vi "TLB Native Dynamic Events ver 0.07D.vi"() -> ()   [LabVIEW 2018]
uses:
  Labview Training Phase 2/Enum Controls/States for Action Engine.ctl
  Type def/TLB event states.ctl
  Type def/TLB MHL States.ctl
  <vilib>/Studica/Studica Toolkit/Background/I2C Channel.ctl
  <vilib>/Studica/Studica Toolkit/NavX/NavX.lvlib
  <vilib>/myRIO/Common/Instrument Driver Framework/myRIO v1.0/AI/typedefs/AI Channels Enum.ctl
  <vilib>/myRIO/Common/Instrument Driver Framework/myRIO v1.0/AI/typedefs/AI Channels List.ctl
  Type def/Type def.ctl
  Type def/Motor Control Cluster.ctl
  <vilib>/Studica/Studica Blackhawk/Blackhawk.lvlib
  <vilib>/Studica/Studica Toolkit/Background/Mxp Selection.ctl
  <vilib>/Studica/Studica Toolkit/Background/DIO Channel.ctl
  <vilib>/NI_Real-Time Target Support.lvlib
  <vilib>/ptbypt/NI_PtbyPt.lvlib
  <vilib>/addons/control/pid/NI_PID_pid.lvlib
  Underlying VI's/Webcam FGV Low level ver/State control.ctl
  <vilib>/userdefined/High Color/IMAQdx.ctl
  <vilib>/addons/control/pid/pid.llb/PID (DBL).vi
panel:
  out "Manual Zero Yaw":bool
  out "BH Loop":i32
  out "NavX Loop":i32
  out "IR Loop":i32
  out "Speed and distance cluster":T1
  out "Cluster":T2
  out "Displacement":T3
  out "Fused Heading":dbl
  in  "error in (no error)":errorcluster
  in  "RED LED State":enum16{"OFF", "ON", "BLINK"}(ring)
  in  "GREEN LED State":enum16{"OFF", "ON", "BLINK"}(ring)
  in  "Red LED":bool
  in  "Green LED":bool
  in  "NavX Zero Yaw":bool
  out "Input state":i8
  out "Waveform Chart 2":dbl(graph)
  out "Waveform Chart":dbl(graph)
  in  "STOP":bool
  out "DIO 0":bool
  out "DIO 1":bool
  out "Limit Switch Array":bool[](array[boolean])
  out "error out":errorcluster
  out "L/R average":fxp<+,64,64>
  out "Right Ultrasonic":fxp<+,64,16>
  out "Left Ultrasonic":fxp<+,64,16>
  out "Right IR Sensor":dbl
  out "Left IR Sensor":dbl
  out "Object detection count":T4
  out "Camera error":errorcluster
  in  "Servo Angle":u8(slide) scale=0.0..180.0
  in  "On/Off":bool
  out "Error":errorcluster
  out "element":T5
  out "Action Queue Items":i32
  out "State Logic Queue Items":i32
  out "Action Queues items":string[](array[string])=["Hardware reset", "Software reset", ""]
  out "State logic":T6=enum."Task 2"
  out "Action State":string
  out "Yaw":dbl
  # "TLB FRAMEWORK STATUS"
  # "Camera Status Loop"
  # "Test Programme written by Calvin Loke    Dated: 28 Aug 2019\nTest Programme revised by Dr Alex See   Dated 30 Aug 2019\n\nProgramme version:   TLB Native Dynamic Events ver 0.04b.vi"
  # "Motor Control Loop"
  # "NAVX Control Loop"
  # "Blackhawk status"
  # "Sensor data"
  # "System Health Status Update"
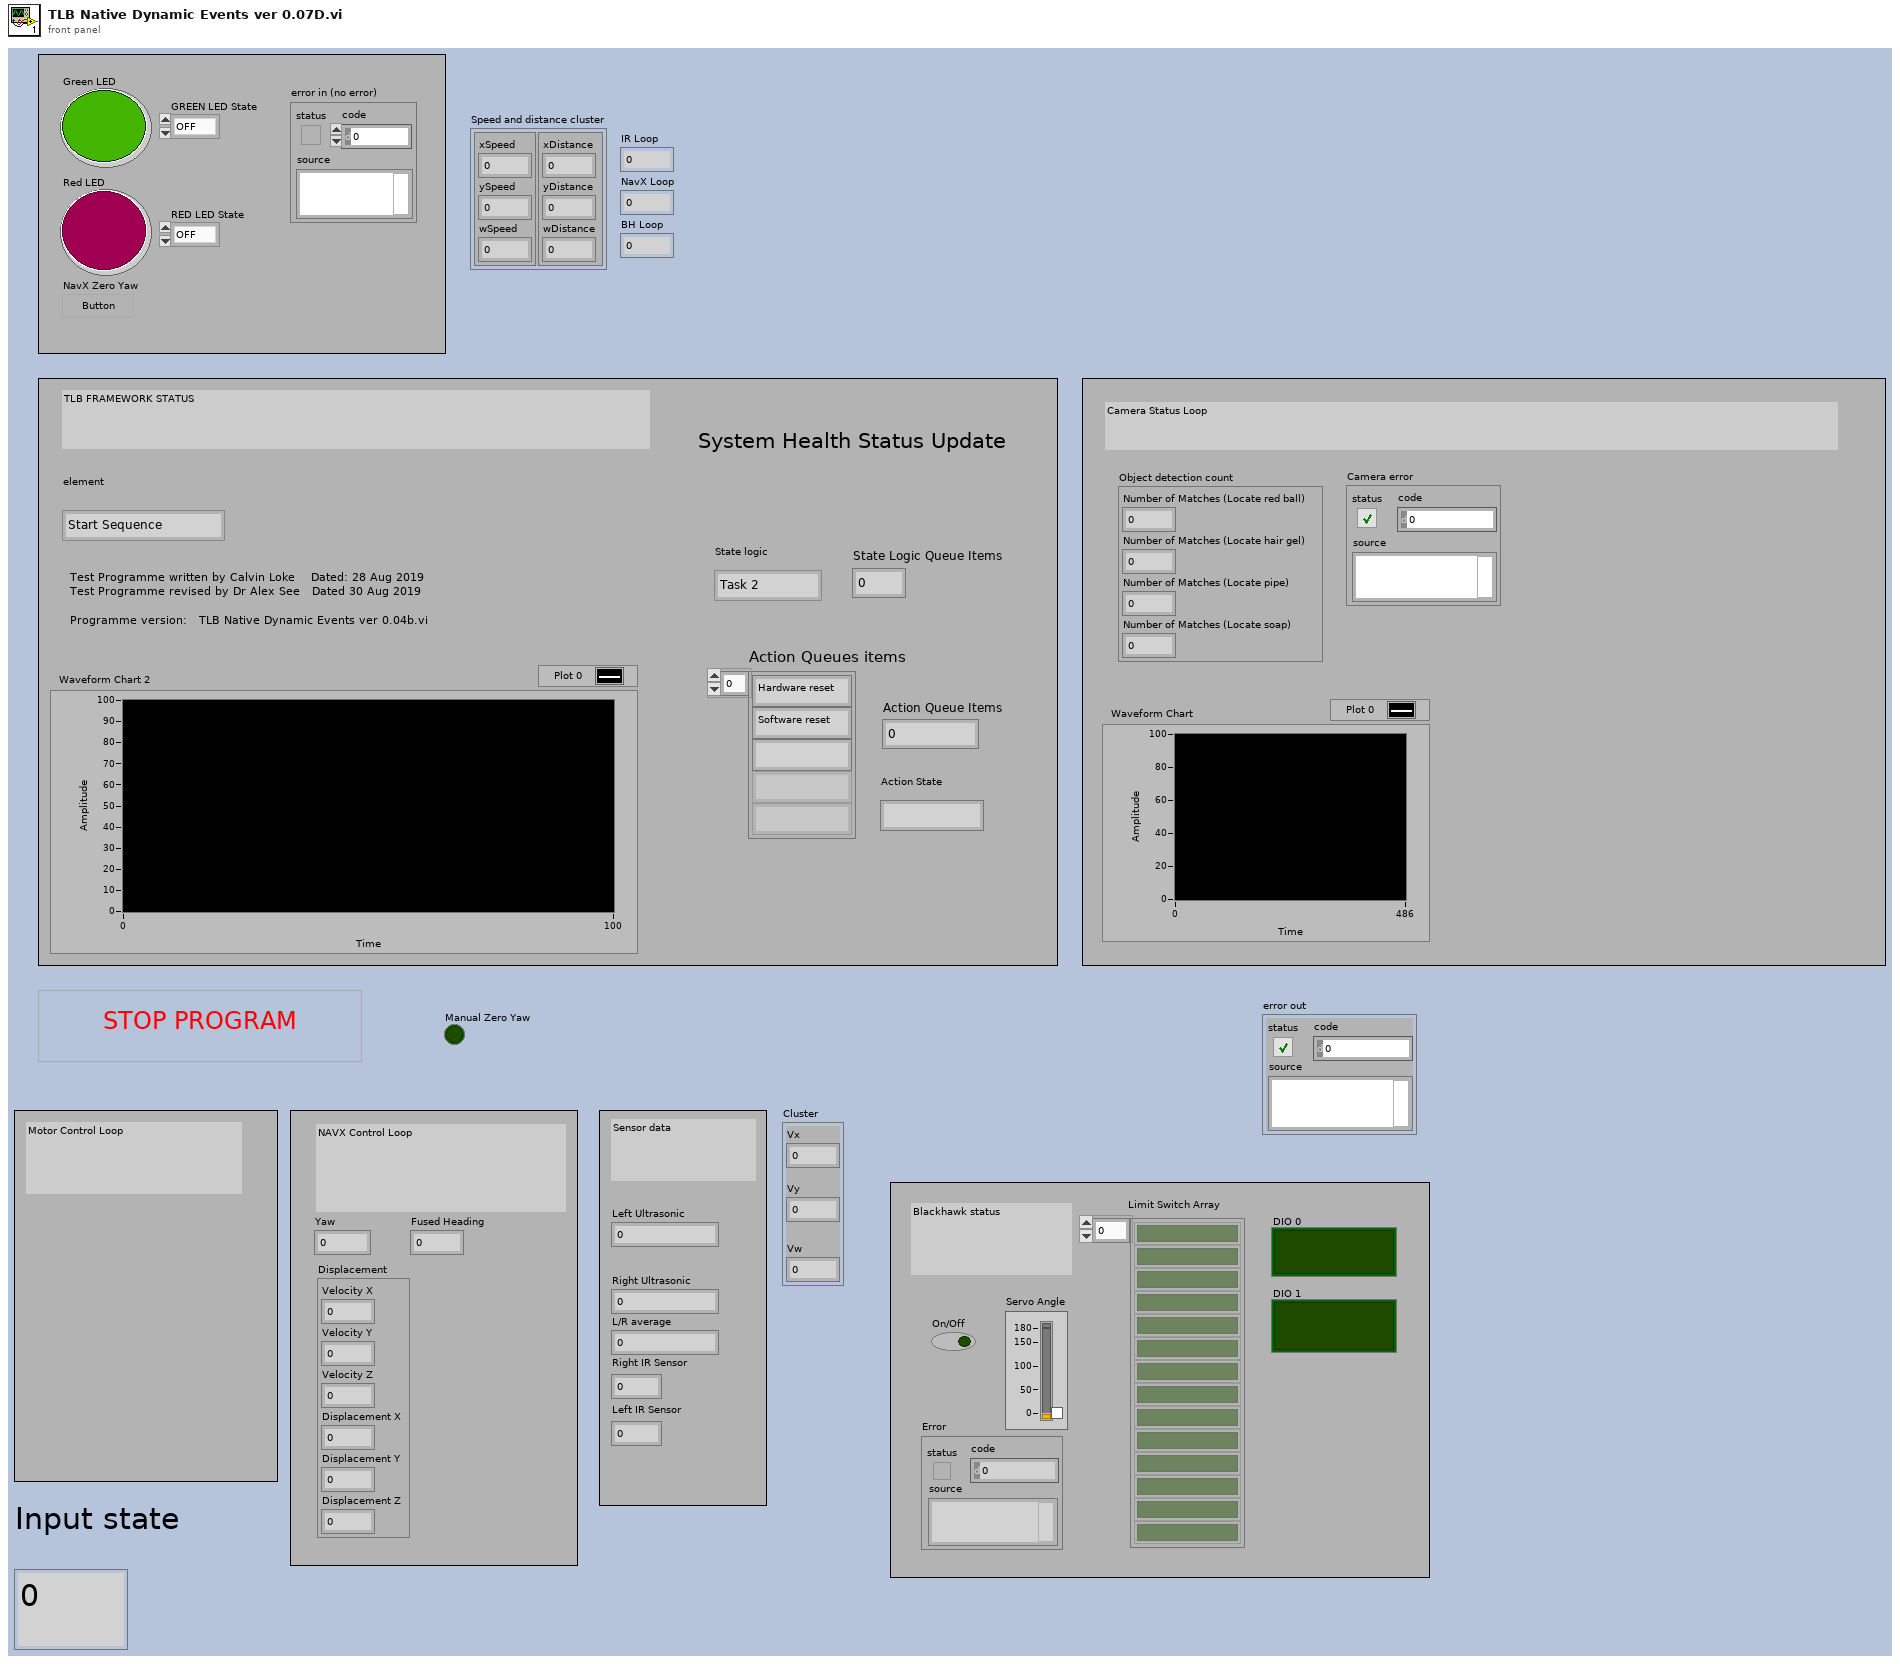
[diagram p1: front panel]
types:
  T1 = cluster{cluster{"xSpeed":dbl, "ySpeed":dbl, "wSpeed":dbl}, cluster{"xDistance":dbl, "yDistance":dbl, "wDistance":dbl}}
  T2 = typedef "Motor Control Cluster.ctl" = cluster{"Vx":dbl, "Vy":dbl, "Vw":dbl}
  T3 = cluster{"Velocity X":dbl, "Velocity Y":dbl, "Velocity Z":dbl, "Displacement X":dbl, "Displacement Y":dbl, "Displacement Z":dbl}
  T4 = cluster{"Number of Matches (Locate red ball)":i32, "Number of Matches (Locate hair gel)":i32, "Number of Matches (Locate pipe)":i32, "Number of Matches (Locate soap)":i32}
  T5 = typedef "TLB event states.ctl" = enum16{"Start Sequence", "Exit", "Start Task 1", "Start Task 2", "Start Task 3", "Start Task 4", "Camera vision", "Wall follow mode", "Idle", "Start Drive Straight"}
  T6 = typedef "TLB MHL States.ctl" = enum16{"None", "Startup", "Idle", "Processing", "Shutdown", "Reset", "Task 1", "Task 2", "Task 3", "Task 4", "Task 4a", "Task 4b", "Task 4c", "Task 4d", "Task 4e", "Task 4f", "Task 4g", "Task 4h", "Acquire image", "Wall follow mode", "Autodrive", "Autodrive a"}
  T7 = typedef "States for Action Engine.ctl" = enum16{"Initialize", "Write", "Read"}
  T8 = typedef "DIO Channel.ctl" = enum16{"Not Connected", "A/DIO1", "A/DIO2", "A/DIO3", "A/DIO4", "A/DIO5", "A/DIO6", "A/DIO7", "A/DIO13", "B/DIO1", "B/DIO2", "B/DIO3", "B/DIO4", "B/DIO5", "B/DIO6", "B/DIO7", "B/DIO13", "C/DIO0", "C/DIO1", "C/DIO2", "C/DIO3", "C/DIO4", "C/DIO5", "C/DIO6", "C/DIO7"}
  T9 = typedef "Type def.ctl" = cluster{"Front Ultrasonic Obstruct":bool, "Left Ultrasonic Obstruct":bool, "Right Ultrasonic Obstruct ":bool}
  T10 = typedef "I2C Channel.ctl" = enum16{"Not Connected", "A", "B"}
  T11 = typedef "TLB MHL States.ctl" = enum16{"None", "Startup", "Idle", "Processing", "Shutdown", "Reset", "Task 1", "Task 2", "Task 3", "Task 4", "Task 4a", "Task 4b", "Task 4c", "Task 4d", "Task 4e", "Task 4f", "Task 4g", "Task 4h", "Acquire image", "Wall follow mode", "Drive Straight"}
  T12 = cluster{"proportional gain (Kc)":dbl, "integral time (Ti, min)":dbl, "derivative time (Td, min)":dbl}
  T13 = typedef "State control.ctl" = enum16{"Initialise", "Start camera", "Continuous Acquisition ", "Stop camera", "Dispose all"}
  T14 = typedef "IMAQdx.ctl" = refnum<k21>
  T15 = typedef "Mxp Selection.ctl" = enum16{"MXP A", "MXP B"}
  T16 = cluster{"xTargetSpeed":dbl, "yTargetSpeed":dbl, "wTargetSpeed":dbl}
  T17 = typedef "AI Channels List.ctl" = T18[]
  T18 = typedef "AI Channels Enum.ctl" = enum16{"Not Connected", "AudioIn/Left", "AudioIn/Right", "C/AI0", "C/AI1", "A/AI0", "A/AI1", "A/AI2", "A/AI3", "A/AI4", "A/AI5", "A/AI6", "A/AI7", "B/AI0", "B/AI1", "B/AI2", "B/AI3", "B/AI4", "B/AI5", "B/AI6", "B/AI7", "AI/AI0", "AI/AI1", "AI/AI2", "AI/AI3", "A/AI0 (DIFF)", "A/AI1 (DIFF)", "A/AI2 (DIFF)", "A/AI3 (DIFF)", "B/AI0 (DIFF)", "B/AI1 (DIFF)", "B/AI2 (DIFF)", "B/AI3 (DIFF)"}
  T19 = cluster{"DIO Channel":T8, "FPGA VI Reference Out":refnum<k20>}
  T20 = typedef "Analog Scaling Constants List.ctl" = T21[]
  T21 = typedef "Analog Scaling Constants.ctl" = cluster{"LSB Weight (Volts)":dbl, "Offset (Volts)":dbl, "Signed?":bool}
  T22 = cluster{"Scale Constants Array":T20, "FPGA Reference Out":refnum<k20>, "AI Channel":T17}
  T23 = cluster{"I2C Channel":T10, "FPGA VI Reference Out":refnum<k20>}
  T24 = typedef "NI_Real-Time Target Support.lvlib/RT CPU Load.ctl" = cluster{"Total (%)":dbl, "Time Critical (%)":dbl, "Timed Structures (%)":dbl, "High (%)":dbl, "Above Normal (%)":dbl, "Normal (%)":dbl, "Background (%)":dbl, "Idle (%)":dbl, "ISR (%)":dbl}
  T25 = cluster{"CPU loads[0]":T24, "CPU loads[1]":T24, "CPU loads[2]":T24, "CPU loads[3]":T24, "CPU loads[4]":T24, "CPU loads[5]":T24, "CPU loads[6]":T24, "CPU loads[7]":T24, "CPU loads[8]":T24}
  T26 = cluster{"I2C Ref Out":cluster{"I2C Channel":T10, "FPGA VI Reference Out":refnum<k20>}, "Connected":bool, "Slave Address (7-bit)":u8, "Registry":u8[]}
  T27 = cluster{"Yaw":dbl, "Roll":dbl, "Pitch":dbl, "Heading":dbl, "Fused Heading":dbl}
  T28 = typedef "IMAQ Image.ctl" = refnum<image>
  T29 = cluster{"xDistance":dbl, "yDistance":dbl, "wDistance":dbl}
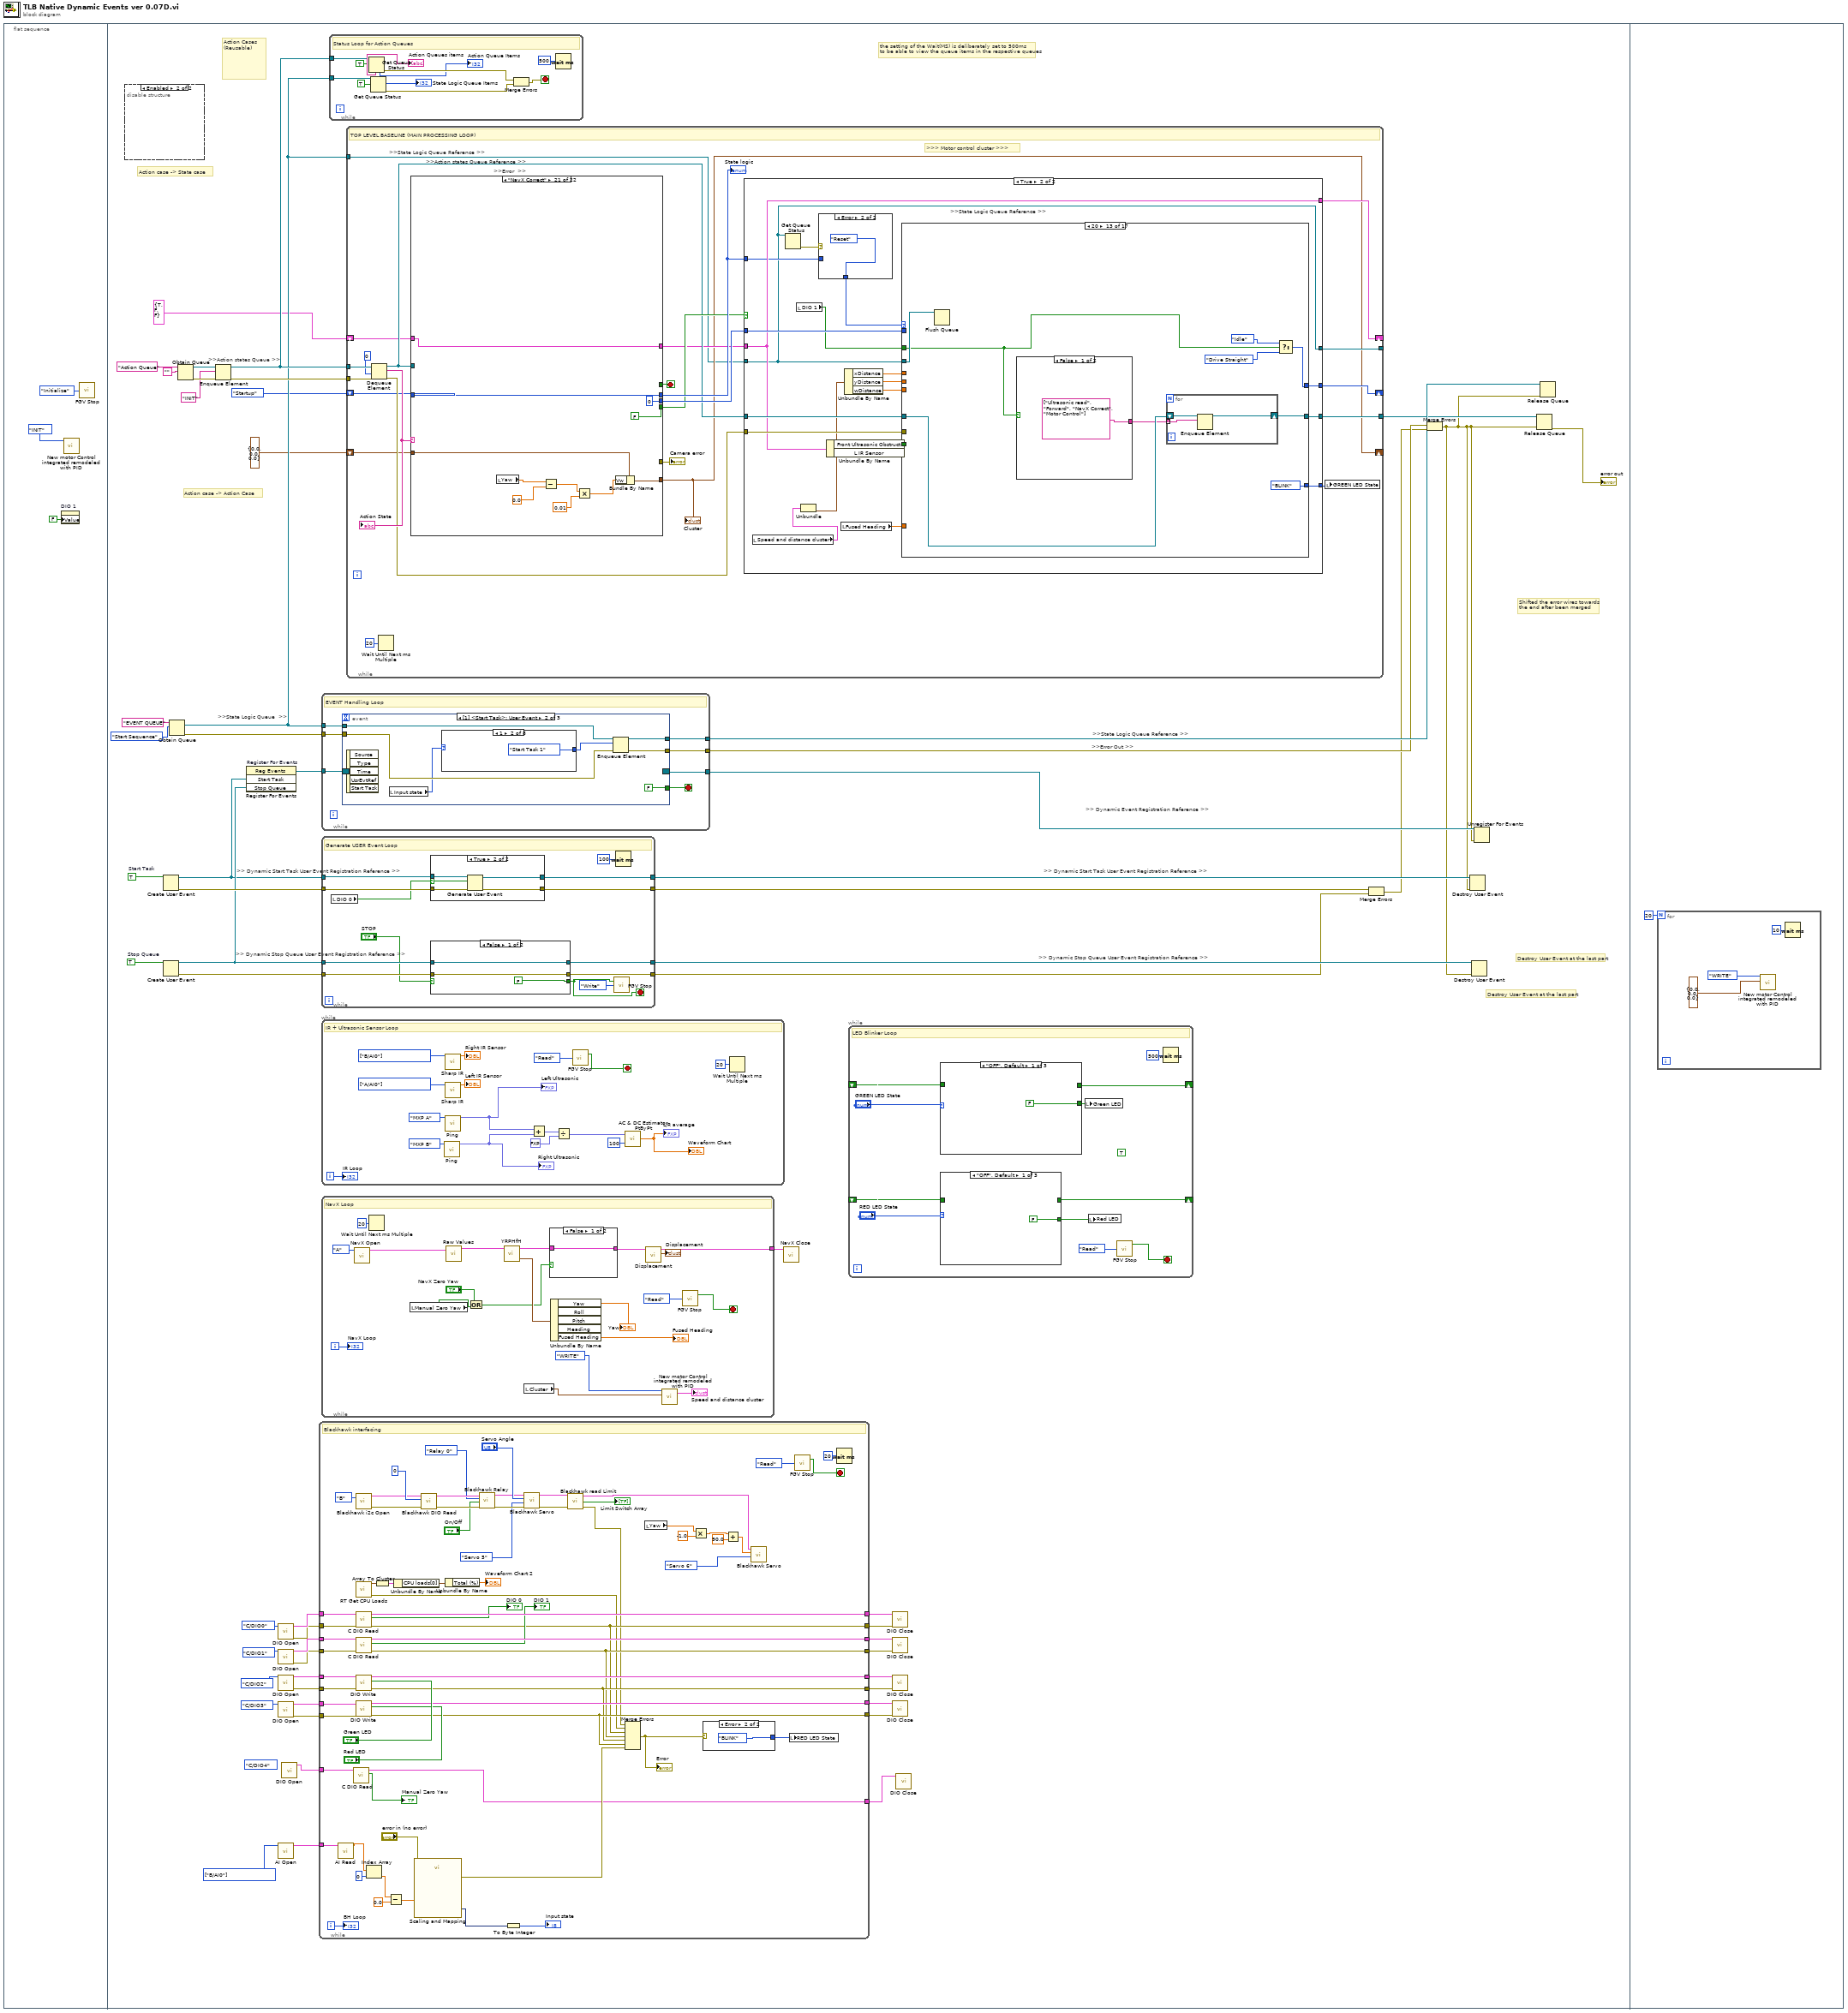
[diagram p0: block diagram]
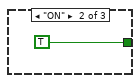
[diagram p2: hidden frame]
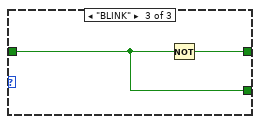
[diagram p3: hidden frame]
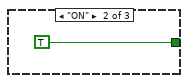
[diagram p4: hidden frame]
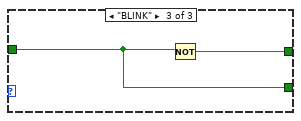
[diagram p5: hidden frame]
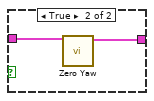
[diagram p6: hidden frame]
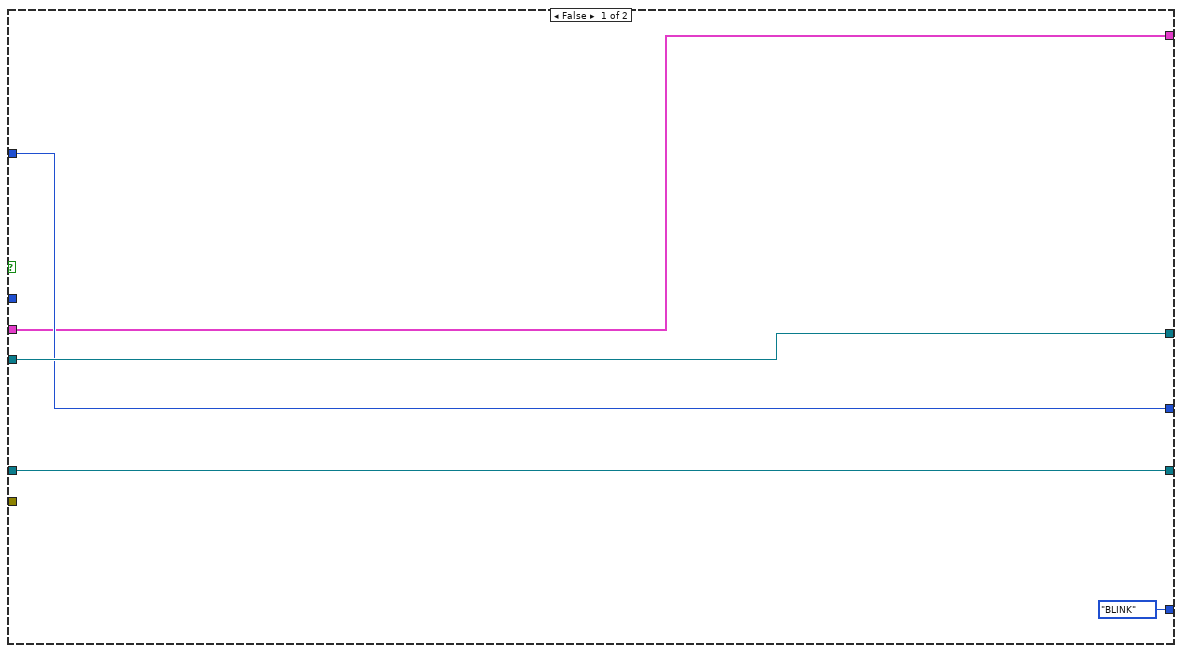
[diagram p7: hidden frame]
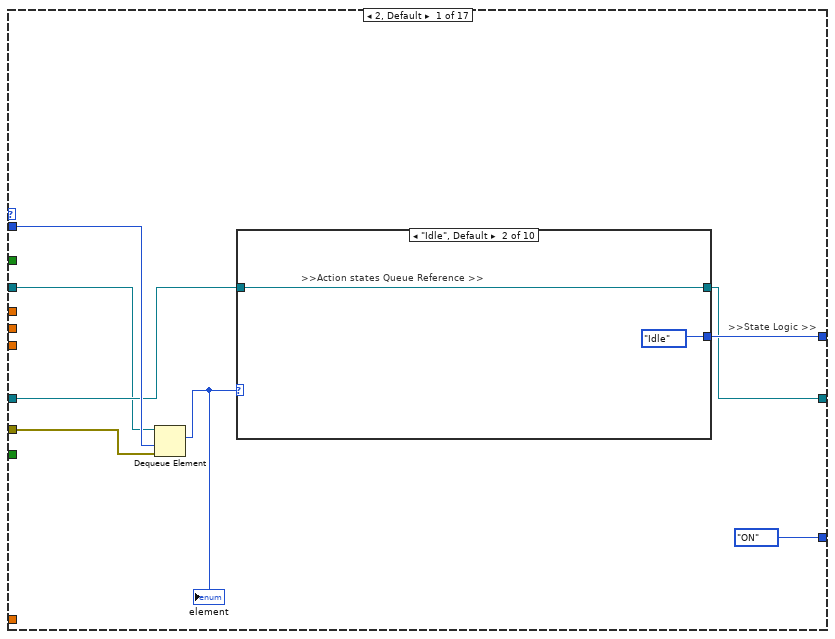
[diagram p9: hidden frame]
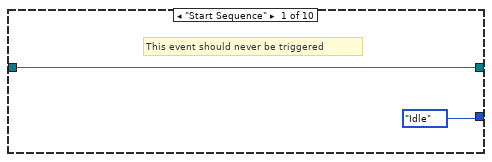
[diagram p10: hidden frame]
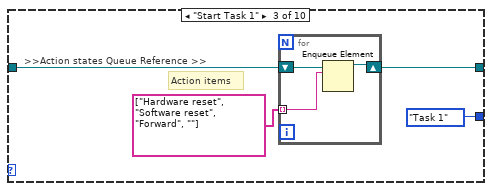
[diagram p11: hidden frame]
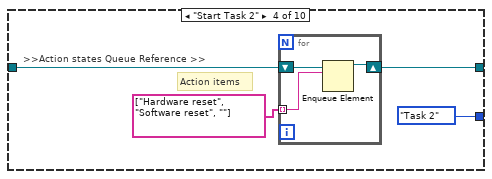
[diagram p12: hidden frame]
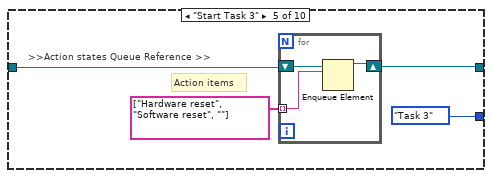
[diagram p13: hidden frame]
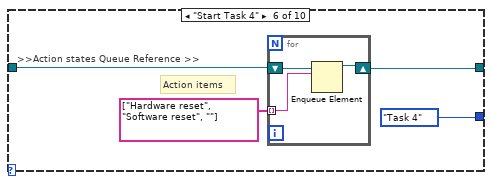
[diagram p14: hidden frame]
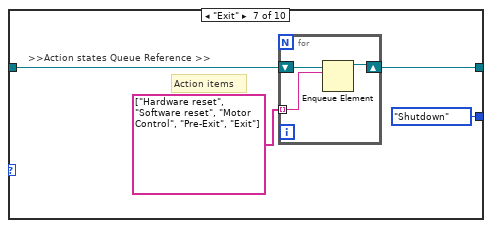
[diagram p15: hidden frame]
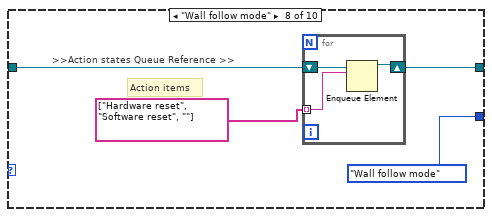
[diagram p16: hidden frame]
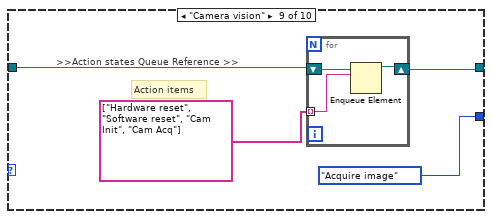
[diagram p17: hidden frame]
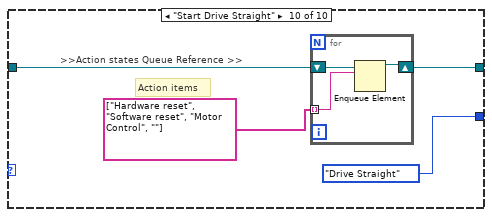
[diagram p18: hidden frame]
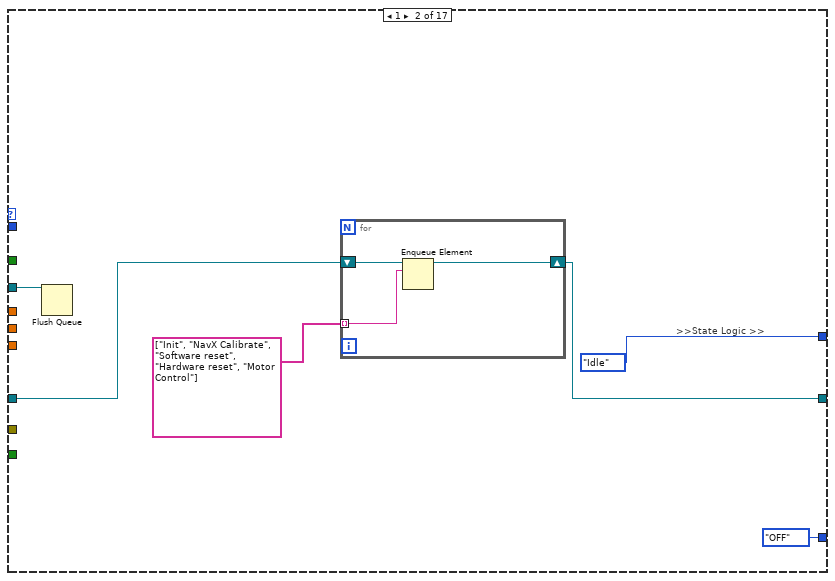
[diagram p19: hidden frame]
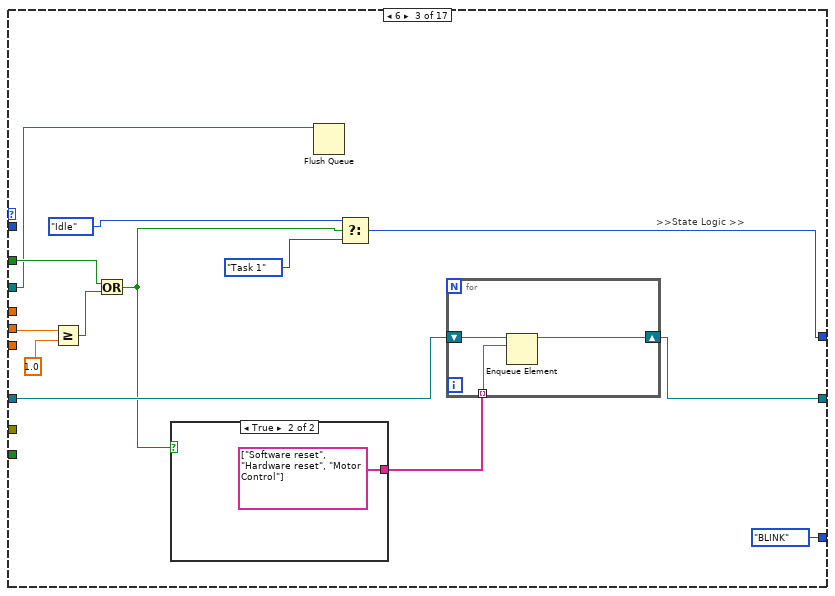
[diagram p20: hidden frame]
diagram:
  n1 = flat-sequence {
    frame #0 {
      n2 = property on="DIO 1" class="Bool (strict)"("Value"=FALSE ("DIO 1")) -> ()  [unwired: 2 in, 2 out]
      n3 = call "New motor Control integrated remodeled with PID.vi"("States"=enum16{"RESET ENCODER", "WRITE", "READ", "INIT"}."INIT") -> ()  [unwired: 4 in, 2 out]
      n4 = call "FGV Stop.vi"("Init/Read/Write State"=States_for_Action_Engine."Initialize") -> ()  [unwired: 2 in, 2 out]
    }
    frame #1 {
      (unwired) DIO_Channel."C/DIO4" ("DIO Channel")
      w11 = T17 [enum."B/AI0"] items=["Not Connected", "AudioIn/Left", "AudioIn/Right", "C/AI0", "C/AI1", "A/AI0", "A/AI1", "A/AI2", "A/AI3", "A/AI4", "A/AI5", "A/AI6", "A/AI7", "B/AI0", "B/AI1", "B/AI2", "B/AI3", "B/AI4", "B/AI5", "B/AI6", "B/AI7", "AI/AI0", "AI/AI1", "AI/AI2", "AI/AI3", "A/AI0 (DIFF)", "A/AI1 (DIFF)", "A/AI2 (DIFF)", "A/AI3 (DIFF)", "B/AI0 (DIFF)", "B/AI1 (DIFF)", "B/AI2 (DIFF)", "B/AI3 (DIFF)"] ("AI Channel")
      w60 = TRUE  # Stop Queue
      w59 = TRUE  # Start Task
      # "Action case -> Action Case"
      # "Action case -> State case"
      # "the setting of the Wait(MS) is deliberately set to 500ms\nto be able to view the queue items in the respective queues"
      # "Action Cases\n(Reusable)"
      # ">>Error Out >>"
      # ">> Dynamic Stop Queue User Event Registration Reference >>"
      # ">> Dynamic Start Task User Event Registration Reference >>"
      # ">> Dynamic Stop Queue User Event Registration Reference >>"
      # ">> Dynamic Start Task User Event Registration Reference >>"
      # ">> Dynamic Event Registration Reference >>"
      # ">>Action states Queue >>"
      # ">>State Logic Queue  >>"
      # ">>State Logic Queue Reference >>"
      # "Destroy User Event at the last part"
      # "Destroy User Event at the last part"
      # "Shifted the error wires towards\nthe end after been merged"
      n5 = disable-structure shown="Enabled" {
        frame Disabled {
          (unwired) variant
          (unwired) TRUE
          n6 = Variant To Data(type="") -> ()  [unwired: 2 in, 2 out]
        }
        frame Enabled {
        }
      }
      n7 = Create User Event(user event datatype=w59) -> (user event=w51:refnum<user-event>, error out=w56:errorcluster)  [unwired: 1 in]
      n8 = Create User Event(user event datatype=w60) -> (user event=w52:refnum<user-event>, error out=w55:errorcluster)  [unwired: 1 in]
      n9 = Obtain Queue(name (unnamed)="EVENT QUEUE", element data type=TLB_event_states."Start Sequence" ("Enum")) -> (queue out=w36:refnum<queue>, error out=w42:errorcluster)  [unwired: 3 in, 1 out]
      n10 = Obtain Queue(name (unnamed)="Action Queue", element data type="") -> (queue out=w45:refnum<queue>, error out=w41:errorcluster)  [unwired: 3 in, 1 out]
      n11 = Enqueue Element(queue=w45, element="INIT", error in (no error)=w41) -> (queue out=w37:refnum<queue>, error out=w40:errorcluster)  [unwired: 1 in, 1 out]
      n12 = register-events "Register For Events"(w51, w52) -> (reference out=w50:refnum<event-registration>)  [unwired: 2 in, 1 out]
      n13 = call <vilib>:"DIO Open.vi"("DIO Channel"=DIO_Channel."C/DIO0") -> ("error out"=w21:errorcluster, "DIO Info Out"=w27:T19)  [unwired: 9 in]
      n14 = call <vilib>:"DIO Open.vi"("DIO Channel"=DIO_Channel."C/DIO1") -> ("error out"=w19:errorcluster, "DIO Info Out"=w23:T19)  [unwired: 9 in]
      n15 = call <vilib>:"DIO Open.vi"("DIO Channel"=DIO_Channel."C/DIO2") -> ("error out"=w9:errorcluster, "DIO Info Out"=w15:T19)  [unwired: 9 in]
      n16 = call <vilib>:"DIO Open.vi"("DIO Channel"=DIO_Channel."C/DIO3") -> ("error out"=w7:errorcluster, "DIO Info Out"=w14:T19)  [unwired: 9 in]
      n17 = call <vilib>:"AI Open.vi"("AI Channel"=w11) -> ("Analog Info"=w10:T22)  [unwired: 9 in, 1 out]
      n18 = call <vilib>:"DIO Open.vi"() -> ("DIO Info Out"=w5:T19)  [unwired: 10 in, 1 out]
      n19 = while {
        tunnel: w27 -> [w748]
        tunnel: [w747] -> w26
        tunnel: w23 -> [w746]
        tunnel: [w745] -> w22
        tunnel: w21 -> [w744]
        tunnel: [w713] -> w20
        tunnel: w19 -> [w743]
        tunnel: [w714] -> w18
        tunnel: w15 -> [w737]
        tunnel: w14 -> [w736]
        tunnel: [w733] -> w13
        tunnel: [w732] -> w12
        tunnel: w10 -> [w731]
        tunnel: w9 -> [w724]
        tunnel: [w715] -> w8
        tunnel: w7 -> [w723]
        tunnel: [w716] -> w6
        tunnel: w5 -> [w700]
        tunnel: [w698] -> w4
        i -> [w707]
        stop <- w761 stop-if-true
        # "Blackhawk interfacing"
        n20 = call <vilib>:"AI Read.vi"("Analog Info"=w731) -> ("Array"=w727:dbl[])  [unwired: 9 in, 1 out]
        n21 = call <vilib>:"C DIO Read.vi"("DIO Info In in"=w700) -> ("IN"=→"Manual Zero Yaw":bool, "DIO Info In out"=w698:T19)  [unwired: 8 in, 1 out]
        n22 = call <vilib>:"Blackhawk i2c Open.vi"("I2C Channel"=I2C_Channel."B") -> ("I2C Ref Out"=w739:T23, "error out"=w738:errorcluster)  [unwired: 2 in]
        n23 = call <vilib>:"RT Get CPU Loads.vi"() -> ("error out"=w712:errorcluster, "CPU loads"=w718:T24[])  [unwired: 10 in]
        n24 = call <vilib>:"C DIO Read.vi"("error in (no error)"=w744, "DIO Info In in"=w748) -> ("error out"=w713:errorcluster, "IN"=→"DIO 0":bool, "DIO Info In out"=w747:T19)  [unwired: 7 in]
        n25 = call <vilib>:"C DIO Read.vi"("error in (no error)"=w743, "DIO Info In in"=w746) -> ("error out"=w714:errorcluster, "IN"=→"DIO 1":bool, "DIO Info In out"=w745:T19)  [unwired: 7 in]
        n26 = call <vilib>:"DIO Write.vi"("error in (no error)"=w724, "Input"="Green LED", "DIO Info In"=w737) -> ("error out"=w715:errorcluster, "DIO Info Out"=w733:T19)  [unwired: 7 in]
        n27 = call <vilib>:"DIO Write.vi"("error in (no error)"=w723, "Input"="Red LED", "DIO Info In"=w736) -> ("error out"=w716:errorcluster, "DIO Info Out"=w732:T19)  [unwired: 7 in]
        n28 = Index Array(array=w727, index=0) -> (element=w729:dbl)
        n29 = Array To Cluster(array=w718) -> (cluster=w719:T25)
        n30 = Subtract(x=w729, y=0.0) -> (x-y=w730:dbl)
        n31 = Unbundle By Name(w719) -> ("CPU loads[0]"=w720:T24)
        n32 = call "Scaling and Mapping"("error in (no error)"="error in (no error)", "Signals"=w730) -> ("error out"=w717:errorcluster, "Scaled Signals"=w725:dynamicdata)  [unwired: 8 in]
        n33 = call <vilib>:"Blackhawk DIO Read.vi"("I2C Ref In"=w739, "PIN"=u8 0, "error in (no error)"=w738) -> ("I2C Ref Out"=w759:T23, "error out"=w760:errorcluster)  [unwired: 3 in, 1 out]
        n34 = Unbundle By Name(w720) -> ("Total (%)"=→"Waveform Chart 2":dbl)
        n35 = call <vilib>:"Blackhawk Relay.vi"("error in (no error)"=w760, "On/Off"="On/Off", "Relay"=enum8{"Relay 0", "Relay 1", "Relay 2"}."Relay 0", "I2C Ref In"=w759) -> ("error out"=w756:errorcluster, "I2C Ref Out"=w753:T23)  [unwired: 6 in]
        n36 = To Byte Integer(number=w725) -> (8bit integer=→"Input state":i8)
        n37 = call <vilib>:"Blackhawk Servo.vi"("error in (no error)"=w756, "Servo Select"=enum16{"Servo 5", "Servo 6"}."Servo 5", "Servo Angle"="Servo Angle", "I2C Ref In"=w753) -> ("error out"=w751:errorcluster, "I2C Ref Out"=w750:T23)  [unwired: 6 in]
        n38 = call <vilib>:"Blackhawk read Limit.vi"("error in (no error)"=w751, "I2C Ref In"=w750) -> ("error out"=w711:errorcluster, "Limit Switch Array"=→"Limit Switch Array":bool[], "I2C Ref Out"=w706:T23)  [unwired: 1 in]
        n39 = Merge Errors(w711, w712, w713, w714, w715, w716, w717) -> (w710:errorcluster)
        "Error" <- w710
        n40 = local read "Yaw"() -> (w701:dbl)
        n41 = Multiply(x=w701, y=-1.0) -> (x*y=w703:dbl)
        n42 = case shown="Error" w710 {
          tunnel: [enum16{"OFF", "ON", "BLINK"}."OFF" ("RED LED State") enum16{"OFF", "ON", "BLINK"}."BLINK" ("RED LED State")] -> w722
          frame No Error {
          }
          frame Error {
          }
        }
        n43 = Add(x=w703, y=90.0) -> (x+y=w705:dbl)
        n44 = call <vilib>:"Blackhawk Servo.vi"("Servo Select"=enum16{"Servo 5", "Servo 6"}."Servo 6", "Servo Angle"=w705, "I2C Ref In"=w706) -> ()  [unwired: 7 in, 2 out]
        n45 = local write "RED LED State"(w722) -> ()
        n46 = call "FGV Stop.vi"("Init/Read/Write State"=States_for_Action_Engine."Read") -> ("Output node"=w761:bool)  [unwired: 2 in, 1 out]
        n47 = Wait (ms)(milliseconds to wait=u32 20) -> ()  [unwired: 1 out]
        "BH Loop" <- w707
      }
      n48 = while {
        tunnel: w50 -> [w641]
        tunnel: [w640] -> w49
        tunnel: w36 -> [w638]
        tunnel: [w637] -> w48
        tunnel: w42 -> [w636]
        tunnel: [w635] -> w39
        stop <- w639 stop-if-true
        # "EVENT Handling Loop"
        n49 = event shown="[1] <Start Task>: User Event" {
          selector: w641 -> [_ _ _]
          dyn-events: [_ _ _] -> w640
          timeout: _ -> [_ _ _]
          tunnel: [FALSE FALSE w668] -> w639
          tunnel: w638 -> [w646 w653 w666]
          tunnel: [w645 w652 w667] -> w637
          tunnel: w636 -> [w643 w651 w664]
          tunnel: [w642 w650 w663] -> w635
          event Timeout {
            n50 = event-data() -> ()  [unwired: 1 in, 3 out]
            n51 = Enqueue Element(queue=w646, element=TLB_event_states."Idle" ("Enum"), error in (no error)=w643) -> (queue out=w645:refnum<queue>, error out=w642:errorcluster)  [unwired: 1 in, 1 out]
          }
          event User Event {
            n52 = event-data() -> ()  [unwired: 1 in, 5 out]
            n53 = local read "Input state"() -> (w649:i8)
            n54 = case shown="1" w649 {
              tunnel: [TLB_event_states."Idle" ("Enum") TLB_event_states."Start Task 1" ("Enum") TLB_event_states."Start Task 2" ("Enum") TLB_event_states."Start Task 3" ("Enum") TLB_event_states."Start Task 4" ("Enum") TLB_event_states."Wall follow mode" ("Enum") TLB_event_states."Camera vision" ("Enum") TLB_event_states."Start Drive Straight" ("Enum")] -> w648
              frame 0 {
              }
              frame 1 {
              }
              frame 2 {
              }
              frame 3, Default {
              }
              frame 4 {
              }
              frame 5 {
              }
              frame 6 {
              }
              frame 7 {
              }
            }
            n55 = Enqueue Element(queue=w653, element=w648, error in (no error)=w651) -> (queue out=w652:refnum<queue>, error out=w650:errorcluster)  [unwired: 1 in, 1 out]
          }
          event User Event {
            n56 = event-data() -> ("Stop Queue"=w668:bool)  [unwired: 1 in, 4 out]
            n57 = Enqueue Element At Opposite End(queue=w666, element=TLB_event_states."Exit" ("Enum"), error in (no error)=w664) -> (queue out=w667:refnum<queue>, error out=w663:errorcluster)  [unwired: 1 in, 1 out]
          }
        }
      }
      n58 = while {
        tunnel: w51 -> [w680]
        tunnel: w52 -> [w679]
        tunnel: [w678] -> w58
        tunnel: [w677] -> w57
        tunnel: w56 -> [w676]
        tunnel: [w675] -> w54
        tunnel: w55 -> [w674]
        tunnel: [w673] -> w53
        stop <- w671 stop-if-true
        # "Generate USER Event Loop"
        n59 = local read "DIO 0"() -> (w670:bool)
        n60 = case shown="True" w670 {
          selector: w670 -> [_ w692]
          tunnel: w680 -> [w691 w696]
          tunnel: [w691 w695] -> w677
          tunnel: w676 -> [w690 w694]
          tunnel: [w690 w693] -> w675
          frame False {
          }
          frame True {
            n61 = Generate User Event(user event=w696, event data cluster=w692, error in=w694) -> (user event out=w695:refnum<user-event>, error out=w693:errorcluster)  [unwired: 1 in]
          }
        }
        n62 = case shown="False" "STOP" {
          selector: "STOP" -> [_ w685]
          tunnel: w679 -> [w684 w689]
          tunnel: [w684 w688] -> w678
          tunnel: w674 -> [w683 w687]
          tunnel: [w683 w686] -> w673
          tunnel: [FALSE w685] -> w671
          frame False {
          }
          frame True {
            n63 = Generate User Event(user event=w689, event data cluster=w685, error in=w687) -> (user event out=w688:refnum<user-event>, error out=w686:errorcluster)  [unwired: 1 in]
          }
        }
        n64 = call "FGV Stop.vi"("Init/Read/Write State"=States_for_Action_Engine."Write", "Input Node"=w671) -> ()  [unwired: 1 in, 2 out]
        n65 = Wait (ms)(milliseconds to wait=u32 100) -> ()  [unwired: 1 out]
      }
      n66 = while {
        i -> [w607]
        stop <- w617 stop-if-true
        w622 = T17 [enum."A/AI0"] items=["Not Connected", "AudioIn/Left", "AudioIn/Right", "C/AI0", "C/AI1", "A/AI0", "A/AI1", "A/AI2", "A/AI3", "A/AI4", "A/AI5", "A/AI6", "A/AI7", "B/AI0", "B/AI1", "B/AI2", "B/AI3", "B/AI4", "B/AI5", "B/AI6", "B/AI7", "AI/AI0", "AI/AI1", "AI/AI2", "AI/AI3", "A/AI0 (DIFF)", "A/AI1 (DIFF)", "A/AI2 (DIFF)", "A/AI3 (DIFF)", "B/AI0 (DIFF)", "B/AI1 (DIFF)", "B/AI2 (DIFF)", "B/AI3 (DIFF)"] ("AI Channel")
        w623 = T17 [enum."B/AI0"] items=["Not Connected", "AudioIn/Left", "AudioIn/Right", "C/AI0", "C/AI1", "A/AI0", "A/AI1", "A/AI2", "A/AI3", "A/AI4", "A/AI5", "A/AI6", "A/AI7", "B/AI0", "B/AI1", "B/AI2", "B/AI3", "B/AI4", "B/AI5", "B/AI6", "B/AI7", "AI/AI0", "AI/AI1", "AI/AI2", "AI/AI3", "A/AI0 (DIFF)", "A/AI1 (DIFF)", "A/AI2 (DIFF)", "A/AI3 (DIFF)", "B/AI0 (DIFF)", "B/AI1 (DIFF)", "B/AI2 (DIFF)", "B/AI3 (DIFF)"] ("AI Channel")
        # "IR + Ultrasonic Sensor Loop"
        n67 = call <vilib>:"Ping.vi"("Mxp Side"=Mxp_Selection."MXP B") -> ("CM"=w611:fxp<+,64,16>)  [unwired: 8 in, 2 out]
        "Right Ultrasonic" <- w611
        n68 = call <vilib>:"Ping.vi"("Mxp Side"=Mxp_Selection."MXP A") -> ("CM"=w612:fxp<+,64,16>)  [unwired: 8 in, 2 out]
        "Left Ultrasonic" <- w612
        n69 = call <vilib>:"Sharp IR.vi"("AI Channel"=w623) -> ("Sharp IR Distance"=→"Right IR Sensor":dbl)  [unwired: 8 in, 2 out]
        n70 = call <vilib>:"Sharp IR.vi"("AI Channel"=w622) -> ("Sharp IR Distance"=→"Left IR Sensor":dbl)  [unwired: 8 in, 2 out]
        n71 = Add(x=w612, y=w611) -> (x+y=w614:fxp<+,64,17>)
        n72 = Divide(x=w614, y=fxp<+,64,17> 2.0) -> (x/y=w610:fxp<+,64,64>)
        n73 = call "FGV Stop.vi"("Init/Read/Write State"=States_for_Action_Engine."Read") -> ("Output node"=w617:bool)  [unwired: 2 in, 1 out]
        n74 = call <vilib>:"AC & DC Estimator PtByPt.vi"("signal"=w610, "sample length"=100) -> ("DC estimate (V)"=→"L/R average" →"Waveform Chart":dbl)  [unwired: 1 in, 2 out]
        n75 = Wait Until Next ms Multiple(millisecond multiple=u32 20) -> ()  [unwired: 1 out]
        "IR Loop" <- w607
      }
      n76 = while {
        tunnel: [w90] -> w28
        i -> [w87]
        stop <- w98 stop-if-true
        # "NavX Loop"
        n77 = call <vilib>:"NavX Open.vi"("I2C Channel"=I2C_Channel."A") -> ("NavX Info"=w92:T26)  [unwired: 9 in, 1 out]
        n78 = Wait Until Next ms Multiple(millisecond multiple=u32 20) -> ()  [unwired: 1 out]
        n79 = local read "Manual Zero Yaw"() -> (w86:bool)
        n80 = call <vilib>:"Raw Values.vi"("NavX Info In"=w92) -> ("NavX Info Out"=w95:T26)  [unwired: 8 in, 1 out]
        n81 = Or(x="NavX Zero Yaw", y=w86) -> (x .or. y?=w84:bool)
        n82 = call <vilib>:"YRPHfH.vi"("NavX Info In"=w95) -> ("YRPHfH"=w96:T27, "NavX Info Out"=w94:T26)  [unwired: 3 in]
        n83 = local read "Cluster"() -> (w80:T2)
        n84 = case shown="False" w84 {
          tunnel: [w100 w102] -> w91
          tunnel: w94 -> [w100 w101]
          frame False {
          }
          frame True {
            n85 = call <vilib>:"Zero Yaw.vi"("NavX Info In"=w101) -> ("NavX Info Out"=w102:T26)  [unwired: 10 in]
          }
        }
        n86 = Unbundle By Name(w96) -> ("Yaw"=→"Yaw":dbl, "Fused Heading"=→"Fused Heading":dbl)  [unwired: 3 out]
        n87 = call <vilib>:"Displacement.vi"("NavX Info In"=w91) -> ("Displacement"=→"Displacement":T3, "NavX Info Out"=w90:T26)  [unwired: 9 in]
        n88 = call "New motor Control integrated remodeled with PID.vi"("States"=enum16{"RESET ENCODER", "WRITE", "READ", "INIT"}."WRITE", "Target Speed"=w80) -> ("Speed and distance cluster"=→"Speed and distance cluster":T1)  [unwired: 3 in, 1 out]
        n89 = call "FGV Stop.vi"("Init/Read/Write State"=States_for_Action_Engine."Read") -> ("Output node"=w98:bool)  [unwired: 2 in, 1 out]
        "NavX Loop" <- w87
      }
      n90 = while {
        tunnel: w37 -> [w632]
        tunnel: w36 -> [w629]
        stop <- w626 stop-if-true
        # "Status Loop for Action Queues"
        n91 = Get Queue Status(queue=w632, return elements? (F)=TRUE) -> (error out=w628:errorcluster, # elements in queue=→"Action Queue Items":i32, elements=→"Action Queues items":string[])  [unwired: 1 in, 5 out]
        n92 = Get Queue Status(queue=w629, return elements? (F)=TRUE) -> (# pending remove=→"State Logic Queue Items":i32, error out=w627:errorcluster)  [unwired: 1 in, 6 out]
        n93 = Merge Errors(w628, w627) -> (w626:errorcluster)
        n94 = Wait (ms)(milliseconds to wait=u32 500) -> ()  [unwired: 1 out]
      }
      n95 = while {
        tunnel: w36 -> [w106]
        shift-right: [w119] -> _
        shift-left: TLB_MHL_States."Startup" ("Enum") -> [w113]
        tunnel: w37 -> [w124]
        tunnel: w40 -> [w122]
        tunnel: [w121] -> _
        tunnel: [w120] -> w31
        shift-right: [w110] -> _
        shift-left: T9 {"Front Ultrasonic Obstruct"=TRUE, "Left Ultrasonic Obstruct"=FALSE, "Right Ultrasonic Obstruct "=FALSE} -> [w112]
        shift-right: [w108] -> _
        shift-left: T2 {"Vx"=0.0, "Vy"=0.0, "Vw"=0.0} -> [w109]
        stop <- w104 stop-if-true
        # ">>> Motor control cluster >>>"
        # ">>Error  >>"
        # ">>Action states Queue Reference >>"
        # ">>State Logic Queue Reference >>"
        # "TOP LEVEL BASELINE (MAIN PROCESSING LOOP)"
        n96 = Dequeue Element(queue=w124, timeout in ms (-1)=0, error in (no error)=w122) -> (queue out=w114:refnum<queue>, element=w123:string, error out=w115:errorcluster)  [unwired: 1 out]
        "Action State" <- w123
        n97 = Wait Until Next ms Multiple(millisecond multiple=u32 20) -> ()  [unwired: 1 out]
        n98 = case shown="\"NavX Correct\"" w123 {
          tunnel: [w424 w436 w443 w451 w460 w468 w474 w484 w491 w496 w506 w515 TLB_MHL_States."Shutdown" ("Enum") w525 w535 w539 w554 w566 w574 w588 w597 w603] -> w125
          tunnel: [w428 0 0 0 0 0 0 0 0 0 0 0 0 0 0 0 0 0 0 0 0 0] -> w118
          tunnel: [TRUE FALSE FALSE FALSE FALSE FALSE FALSE FALSE FALSE FALSE FALSE FALSE FALSE FALSE FALSE FALSE FALSE FALSE FALSE FALSE FALSE FALSE] -> w117
          tunnel: w114 -> [_ _ _ _ _ _ _ _ _ _ _ _ _ _ _ _ _ _ _ _ _ _]
          tunnel: w113 -> [w424 w436 w443 w451 w460 w468 w474 w484 w491 w496 w506 w515 _ w525 w535 w539 w554 w566 w574 w588 w597 w603]
          tunnel: w112 -> [w426 w433 w440 w448 w456 w464 w472 w480 w488 w497 w503 w511 w518 w526 w534 w542 w555 w567 w573 w584 w595 w605]
          tunnel: [w426 w433 w440 w448 w456 w464 w472 w480 w488 w497 w502 w511 w518 w526 w531 w541 w555 w567 w573 w584 w595 w605] -> w111
          tunnel: w109 -> [w425 w432 w439 w447 w454 w463 w470 w479 w486 w493 w500 w510 w517 w522 w528 w536 w550 w565 w577 w585 w598 w604]
          tunnel: [w425 w432 w437 w445 w455 w462 w471 w478 w487 w493 w500 w508 w517 w522 w528 w536 w551 w565 w577 w585 w599 w604] -> w108
          tunnel: [_ _ _ _ _ _ _ _ _ _ _ _ _ _ _ _ _ w556 w569 w578 _ _] -> w107
          tunnel: [_ _ _ _ _ _ _ _ _ _ _ _ TRUE _ _ _ _ _ _ _ _ _] -> w104
          frame "No action", Default {
            n99 = case shown="1, Default" w424 {
              tunnel: [0 100] -> w428
              frame 1, Default {
              }
              frame 2 {
              }
            }
            n100 = local write "NavX Zero Yaw"(FALSE ("NavX Zero Yaw")) -> ()
          }
          frame "Init" {
            # ">>State Logic  >>"
            n101 = local write "Servo Angle"(u8 90 ("Servo Angle")) -> ()
          }
          frame "Forward" {
            n102 = local write "NavX Zero Yaw"(FALSE ("NavX Zero Yaw")) -> ()
            n103 = Bundle By Name(cluster=w439, "Vy"=0.6) -> (w437:T2)
          }
          frame "Reverse" {
            n104 = local write "NavX Zero Yaw"(FALSE ("NavX Zero Yaw")) -> ()
            n105 = Bundle By Name(cluster=w447, "Vy"=-0.6) -> (w445:T2)
          }
          frame "Right" {
            n106 = local write "NavX Zero Yaw"(FALSE ("NavX Zero Yaw")) -> ()
            n107 = Bundle By Name(cluster=w454, "Vx"=0.6) -> (w455:T2)
          }
          frame "Left" {
            n108 = Bundle By Name(cluster=w463, "Vx"=-0.6) -> (w462:T2)
            n109 = local write "NavX Zero Yaw"(FALSE ("NavX Zero Yaw")) -> ()
          }
          frame "Rotate CW" {
            n110 = local write "NavX Zero Yaw"(FALSE ("NavX Zero Yaw")) -> ()
            n111 = Bundle By Name(cluster=w470, "Vw"=-0.3) -> (w471:T2)
          }
          frame "Rotate ACW" {
            n112 = local write "NavX Zero Yaw"(FALSE ("NavX Zero Yaw")) -> ()
            n113 = Bundle By Name(cluster=w479, "Vw"=0.15) -> (w478:T2)
          }
          frame "Stop" {
            w485 = 0.0
            n114 = local write "NavX Zero Yaw"(FALSE ("NavX Zero Yaw")) -> ()
            n115 = Bundle By Name(cluster=w486, "Vx"=w485, "Vy"=w485, "Vw"=w485) -> (w487:T2)
          }
          frame "Motor control" {
          }
          frame "Software reset" {
            w501 = FALSE ("NavX Zero Yaw")
            n116 = Wait (ms)(milliseconds to wait=u32 20) -> ()  [unwired: 1 out]
            n117 = local write "NavX Zero Yaw"(w501) -> ()
            n118 = Bundle By Name(cluster=w503, "Front Ultrasonic Obstruct"=w501, "L IR Sensor"=0.0) -> (w502:T9)
          }
          frame "Hardware reset" {
            w509 = 0.0
            n119 = Wait (ms)(milliseconds to wait=u32 100) -> ()  [unwired: 1 out]
            n120 = local write "NavX Zero Yaw"(TRUE ("NavX Zero Yaw")) -> ()
            n121 = Bundle By Name(cluster=w510, "Vx"=w509, "Vy"=w509, "Vw"=w509) -> (w508:T2)
          }
          frame "Exit" {
          }
          frame "Pre-Exit" {
          }
          frame "Ultrasonic read" {
            # "Object detection"
            n122 = local read "L/R average"() -> (w527:fxp<+,64,64>)
            n123 = Less Or Equal?(x=w527, y=35.0) -> (x <= y?=w529:bool)
            n124 = Bundle By Name(cluster=w534, "Front Ultrasonic Obstruct"=w529) -> (w531:T9)
          }
          frame "IR Sensor Read" {
            n125 = local read "Left IR Sensor"() -> (w540:dbl)
            n126 = Bundle By Name(cluster=w542, "L IR Sensor"=w540) -> (w541:T9)
          }
          frame "Calculate" {
            n127 = Unbundle By Name(w555) -> ("L IR Sensor"=w547:dbl)
            n128 = call-poly <vilib>:"PID.vi"("output range"=cluster{"output high":dbl, "output low":dbl} {"output high"=0.3, "output low"=-0.3}, "PID gains"=T12 {"proportional gain (Kc)"=0.01, "integral time (Ti, min)"=0.0, "derivative time (Td, min)"=0.0}, "process variable"=w547, "setpoint"=20.0) -> ("output"=w544:dbl)  [unwired: 6 in, 1 out]
            n129 = Negate(x=w544) -> (-x=w543:dbl)
            n130 = Bundle By Name(cluster=w550, "Vy"=0.2, "Vw"=w543) -> (w551:T2)
          }
          frame "Cam Init" {
            n131 = call "Low-Level Grab.vi"("States"=State_control."Initialise", "Session In"=T14 "cam1") -> ("error out"=w557:errorcluster, "Session Out"=w558:T14)  [unwired: 7 in, 1 out]
            n132 = call "Low-Level Grab.vi"("error in (no error)"=w557, "States"=State_control."Start camera", "Session In"=w558) -> ("error out"=w556:errorcluster)  [unwired: 6 in, 2 out]
            n133 = local write "Servo Angle"(u8 170 ("Servo Angle")) -> ()
          }
          frame "Cam Acq" {
            n134 = call "Low-Level Grab.vi"("States"=State_control."Continuous Acquisition ") -> ("error out"=w570:errorcluster, "Image Out"=w571:T28)  [unwired: 8 in, 1 out]
            n135 = call "All object detection ver2.vi"("Image In"=w571, "error in"=w570) -> ("Object detection count"=→"Object detection count":T4, "error out"=w569:errorcluster)  [unwired: 1 out]
          }
          frame "Cam Exit" {
            n136 = call "Low-Level Grab.vi"("States"=State_control."Stop camera") -> ("error out"=w579:errorcluster, "Session Out"=w581:T14)  [unwired: 8 in, 1 out]
            n137 = call "Low-Level Grab.vi"("error in (no error)"=w579, "States"=State_control."Dispose all", "Session In"=w581) -> ("error out"=w578:errorcluster)  [unwired: 6 in, 2 out]
            n138 = local write "Servo Angle"(u8 90 ("Servo Angle")) -> ()
          }
          frame "NavX Correct" {
            n139 = local read "Yaw"() -> (w593:dbl)
            n140 = Subtract(x=w593, y=0.0) -> (x-y=w591:dbl)
            n141 = Multiply(x=w591, y=0.01) -> (x*y=w590:dbl)
            n142 = Bundle By Name(cluster=w598, "Vw"=w590) -> (w599:T2)
          }
          frame "NavX Calibrate" {
            n143 = Wait (ms)(milliseconds to wait=u32 1000) -> ()  [unwired: 1 out]
          }
        }
        "State logic" <- w125
        "Camera error" <- w107
        "Cluster" <- w108
        n144 = case shown="True" w117 {
          tunnel: w125 -> [w129 w136]
          tunnel: w106 -> [w130 w135]
          tunnel: w114 -> [w128 w149]
          tunnel: [w130 w135] -> w121
          tunnel: [w128 w148] -> w120
          tunnel: [w129 w147] -> w119
          tunnel: w115 -> [_ w146]
          tunnel: w118 -> [_ w145]
          tunnel: w111 -> [w127 w139]
          tunnel: [w127 w139] -> w110
          tunnel: [enum16{"OFF", "ON", "BLINK"}."BLINK" ("GREEN LED State") w132] -> w103
          frame False {
          }
          frame True {
            # ">>State Logic Queue Reference >>"
            n145 = local read "Speed and distance cluster"() -> (w131:T1)
            n146 = Get Queue Status(queue=w135) -> (error out=w134:errorcluster)  [unwired: 2 in, 7 out]
            n147 = local read "DIO 1"() -> (w133:bool)
            n148 = Unbundle(w131) -> (w138:T29)  [unwired: 1 out]
            n149 = case shown="Error" w134 {
              tunnel: [w150 TLB_MHL_States."Reset" ("Enum")] -> w137
              tunnel: w136 -> [w150 _]
              frame No Error {
              }
              frame Error {
              }
            }
            n150 = Unbundle By Name(w139) -> ("Front Ultrasonic Obstruct"=w140:bool)  [unwired: 1 out]
            n151 = local read "Fused Heading"() -> (w141:dbl)
            n152 = Unbundle By Name(w138) -> ("xDistance"=w142:dbl, "yDistance"=w144:dbl, "wDistance"=w143:dbl)
            n153 = case shown="20" w137 {
              tunnel: w135 -> [w153 w220 w230 w248 w267 w283 w297 w313 w329 w346 _ w370 w386 w398 _ _ _]
              tunnel: w149 -> [w155 w223 w237 w252 w276 w287 w303 w320 w335 w352 w363 w373 w387 w402 w411 w415 w421]
              tunnel: [w154 w222 w236 w253 w275 w288 w302 w319 w334 w351 w362 w374 w388 w401 w411 w414 w421] -> w148
              tunnel: [w158 TLB_MHL_States."Idle" ("Enum") w239 w254 w272 w291 w305 w318 w336 w350 TLB_MHL_States."Shutdown" ("Enum") w376 w389 w400 TLB_MHL_States."Reset" ("Enum") TLB_MHL_States."Shutdown" ("Enum") TLB_MHL_States."Reset" ("Enum")] -> w147
              tunnel: w146 -> [w156 _ _ _ _ _ _ _ _ _ _ _ _ _ _ _ _]
              tunnel: w145 -> [w157 _ _ _ _ _ _ _ _ _ _ _ _ _ _ _ _]
              tunnel: w133 -> [_ _ w234 w251 w270 _ _ _ _ w349 _ w371 w384 w399 _ _ _]
              tunnel: w144 -> [_ _ w231 _ _ _ _ w315 _ _ _ _ _ _ _ _ _]
              tunnel: w143 -> [_ _ _ _ _ _ _ _ _ _ _ _ _ _ _ _ _]
              tunnel: w142 -> [_ _ _ _ _ _ w299 _ w331 _ _ _ _ _ _ _ _]
              tunnel: w141 -> [_ _ _ _ w266 _ _ _ _ _ _ _ _ _ _ _ _]
              tunnel: w140 -> [_ _ _ w249 _ w285 _ _ _ w348 _ _ _ _ _ _ _]
              tunnel: [enum16{"OFF", "ON", "BLINK"}."ON" ("GREEN LED State") enum16{"OFF", "ON", "BLINK"}."OFF" ("GREEN LED State") enum16{"OFF", "ON", "BLINK"}."BLINK" ("GREEN LED State") enum16{"OFF", "ON", "BLINK"}."BLINK" ("GREEN LED State") enum16{"OFF", "ON", "BLINK"}."BLINK" ("GREEN LED State") enum16{"OFF", "ON", "BLINK"}."BLINK" ("GREEN LED State") enum16{"OFF", "ON", "BLINK"}."BLINK" ("GREEN LED State") enum16{"OFF", "ON", "BLINK"}."BLINK" ("GREEN LED State") enum16{"OFF", "ON", "BLINK"}."BLINK" ("GREEN LED State") enum16{"OFF", "ON", "BLINK"}."BLINK" ("GREEN LED State") enum16{"OFF", "ON", "BLINK"}."OFF" ("GREEN LED State") enum16{"OFF", "ON", "BLINK"}."BLINK" ("GREEN LED State") enum16{"OFF", "ON", "BLINK"}."BLINK" ("GREEN LED State") enum16{"OFF", "ON", "BLINK"}."BLINK" ("GREEN LED State") _ enum16{"OFF", "ON", "BLINK"}."OFF" ("GREEN LED State") _] -> w132
              frame 2, Default {
                # ">>State Logic >>"
                n154 = Dequeue Element(queue=w153, timeout in ms (-1)=w157, error in (no error)=w156) -> (element=w159:T5)  [unwired: 3 out]
                "element" <- w159
                n155 = case shown="\"Idle\", Default" w159 {
                  tunnel: [TLB_MHL_States."Idle" ("Enum") TLB_MHL_States."Idle" ("Enum") TLB_MHL_States."Task 1" ("Enum") TLB_MHL_States."Task 2" ("Enum") TLB_MHL_States."Task 3" ("Enum") TLB_MHL_States."Task 4" ("Enum") TLB_MHL_States."Shutdown" ("Enum") TLB_MHL_States."Wall follow mode" ("Enum") TLB_MHL_States."Acquire image" ("Enum") TLB_MHL_States."Drive Straight" ("Enum")] -> w158
                  tunnel: [w161 w162 w166 w171 w180 w186 w192 w199 w207 w214] -> w154
                  tunnel: w155 -> [w161 w162 w164 w172 w181 w187 w193 w200 w208 w215]
                  frame "Start Sequence" {
                    # "This event should never be triggered"
                  }
                  frame "Idle", Default {
                    # ">>Action states Queue Reference >>"
                  }
                  frame "Start Task 1" {
                    # ">>Action states Queue Reference >>"
                    # "Action items"
                    n156 = for {
                      shift-right: [w170] -> w166
                      shift-left: w164 -> [w169]
                      tunnel: string[] ["Hardware reset", "Software reset", "Forward", ""] -> [w168] mode=indexing
                      n157 = Enqueue Element(queue=w169, element=w168) -> (queue out=w170:refnum<queue>)  [unwired: 2 in, 2 out]
                    }
                  }
                  frame "Start Task 2" {
                    # ">>Action states Queue Reference >>"
                    # "Action items"
                    n158 = for {
                      shift-right: [w177] -> w171
                      shift-left: w172 -> [w176]
                      tunnel: string[] ["Hardware reset", "Software reset", ""] -> [w175] mode=indexing
                      n159 = Enqueue Element(queue=w176, element=w175) -> (queue out=w177:refnum<queue>)  [unwired: 2 in, 2 out]
                    }
                  }
                  frame "Start Task 3" {
                    # ">>Action states Queue Reference >>"
                    # "Action items"
                    n160 = for {
                      shift-right: [w184] -> w180
                      shift-left: w181 -> [w183]
                      tunnel: string[] ["Hardware reset", "Software reset", ""] -> [w182] mode=indexing
                      n161 = Enqueue Element(queue=w183, element=w182) -> (queue out=w184:refnum<queue>)  [unwired: 2 in, 2 out]
                    }
                  }
                  frame "Start Task 4" {
                    # ">>Action states Queue Reference >>"
                    # "Action items"
                    n162 = for {
                      shift-right: [w191] -> w186
                      shift-left: w187 -> [w190]
                      tunnel: string[] ["Hardware reset", "Software reset", ""] -> [w189] mode=indexing
                      n163 = Enqueue Element(queue=w190, element=w189) -> (queue out=w191:refnum<queue>)  [unwired: 2 in, 2 out]
                    }
                  }
                  frame "Exit" {
                    # ">>Action states Queue Reference >>"
                    # "Action items"
                    n164 = for {
                      shift-right: [w198] -> w192
                      shift-left: w193 -> [w197]
                      tunnel: string[] ["Hardware reset", "Software reset", "Motor Control", "Pre-Exit", "Exit"] -> [w196] mode=indexing
                      n165 = Enqueue Element(queue=w197, element=w196) -> (queue out=w198:refnum<queue>)  [unwired: 2 in, 2 out]
                    }
                  }
                  frame "Wall follow mode" {
                    # ">>Action states Queue Reference >>"
                    # "Action items"
                    n166 = for {
                      shift-right: [w205] -> w199
                      shift-left: w200 -> [w204]
                      tunnel: string[] ["Hardware reset", "Software reset", ""] -> [w203] mode=indexing
                      n167 = Enqueue Element(queue=w204, element=w203) -> (queue out=w205:refnum<queue>)  [unwired: 2 in, 2 out]
                    }
                  }
                  frame "Camera vision" {
                    # ">>Action states Queue Reference >>"
                    # "Action items"
                    n168 = for {
                      shift-right: [w212] -> w207
                      shift-left: w208 -> [w211]
                      tunnel: string[] ["Hardware reset", "Software reset", "Cam Init", "Cam Acq"] -> [w210] mode=indexing
                      n169 = Enqueue Element(queue=w211, element=w210) -> (queue out=w212:refnum<queue>)  [unwired: 2 in, 2 out]
                    }
                  }
                  frame "Start Drive Straight" {
                    # ">>Action states Queue Reference >>"
                    # "Action items"
                    n170 = for {
                      shift-right: [w219] -> w214
                      shift-left: w215 -> [w218]
                      tunnel: string[] ["Hardware reset", "Software reset", "Motor Control", ""] -> [w217] mode=indexing
                      n171 = Enqueue Element(queue=w218, element=w217) -> (queue out=w219:refnum<queue>)  [unwired: 2 in, 2 out]
                    }
                  }
                }
              }
              frame 1 {
                # ">>State Logic >>"
                n172 = Flush Queue(queue=w220) -> ()  [unwired: 1 in, 3 out]
                n173 = for {
                  shift-right: [w227] -> w222
                  shift-left: w223 -> [w228]
                  tunnel: string[] ["Init", "NavX Calibrate", "Software reset", "Hardware reset", "Motor Control"] -> [w226] mode=indexing
                  n174 = Enqueue Element(queue=w228, element=w226) -> (queue out=w227:refnum<queue>)  [unwired: 2 in, 2 out]
                }
              }
              frame 6 {
                # ">>State Logic >>"
                n175 = Greater Or Equal?(x=w231, y=1.0) -> (x >= y?=w232:bool)
                n176 = Or(x=w234, y=w232) -> (x .or. y?=w235:bool)
                n177 = case shown="True" w235 {
                  tunnel: [string[] ["Forward", "Motor Control", ""] string[] ["Software reset", "Hardware reset", "Motor Control"]] -> w238
                  frame False {
                  }
                  frame True {
                  }
                }
                n178 = Flush Queue(queue=w230) -> ()  [unwired: 1 in, 3 out]
                n179 = Select(t=TLB_MHL_States."Idle" ("Enum"), s=w235, f=TLB_MHL_States."Task 1" ("Enum")) -> (s? t:f=w239:T6)
                n180 = for {
                  shift-right: [w245] -> w236
                  shift-left: w237 -> [w246]
                  tunnel: w238 -> [w244] mode=indexing
                  n181 = Enqueue Element(queue=w246, element=w244) -> (queue out=w245:refnum<queue>)  [unwired: 2 in, 2 out]
                }
              }
              frame 7 {
                # ">>State Logic >>"
                n182 = Flush Queue(queue=w248) -> ()  [unwired: 1 in, 3 out]
                n183 = case shown="True" w251 {
                  tunnel: [w258 string[] ["Hardware reset", "Software reset", "Motor control"]] -> w250
                  tunnel: w249 -> [w257 _]
                  frame False {
                    n184 = case shown="False" w257 {
                      tunnel: [string[] ["Stop", "Ultrasonic read", "Motor Control"] string[] ["Reverse", "Ultrasonic read", "Motor control"]] -> w258
                      frame False {
                      }
                      frame True {
                      }
                    }
                  }
                  frame True {
                  }
                }
                n185 = Select(t=TLB_MHL_States."Idle" ("Enum"), s=w251, f=TLB_MHL_States."Task 2" ("Enum")) -> (s? t:f=w254:T6)
                n186 = for {
                  shift-right: [w263] -> w253
                  shift-left: w252 -> [w264]
                  tunnel: w250 -> [w262] mode=indexing
                  n187 = Enqueue Element(queue=w264, element=w262) -> (queue out=w263:refnum<queue>)  [unwired: 2 in, 2 out]
                }
              }
              frame 8 {
                n188 = Greater Or Equal?(x=w266, y=360.0) -> (x >= y?=w269:bool)
                n189 = Flush Queue(queue=w267) -> ()  [unwired: 1 in, 3 out]
                n190 = Or(x=w269, y=w270) -> (x .or. y?=w271:bool)
                n191 = case shown="False" w271 {
                  tunnel: [string[] ["Rotate CW", "Motor Control"] string[] ["Software reset", "Hardware reset", "Motor Control"]] -> w277
                  frame False {
                  }
                  frame True {
                  }
                }
                n192 = for {
                  shift-right: [w279] -> w275
                  shift-left: w276 -> [w280]
                  tunnel: w277 -> [w278] mode=indexing
                  n193 = Enqueue Element(queue=w280, element=w278) -> (queue out=w279:refnum<queue>)  [unwired: 2 in, 2 out]
                }
                n194 = Select(t=TLB_MHL_States."Idle" ("Enum"), s=w271, f=TLB_MHL_States."Task 3" ("Enum")) -> (s? t:f=w272:T6)
              }
              frame 9 {
                n195 = Flush Queue(queue=w283) -> ()  [unwired: 1 in, 3 out]
                n196 = case shown="True" w285 {
                  tunnel: [string[] ["Forward", "Ultrasonic read", "Motor Control"] string[] ["Stop", "Hardware reset", "Software reset", "Motor Control"]] -> w286
                  frame False {
                  }
                  frame True {
                  }
                }
                n197 = for {
                  shift-right: [w295] -> w288
                  shift-left: w287 -> [w296]
                  tunnel: w286 -> [w294] mode=indexing
                  n198 = Enqueue Element(queue=w296, element=w294) -> (queue out=w295:refnum<queue>)  [unwired: 2 in, 2 out]
                }
                n199 = Select(t=TLB_MHL_States."Task 4a" ("Enum"), s=w285, f=TLB_MHL_States."Task 4" ("Enum")) -> (s? t:f=w291:T6)
              }
              frame 10 {
                n200 = Greater Or Equal?(x=w299, y=0.5) -> (x >= y?=w301:bool)
                n201 = Flush Queue(queue=w297) -> ()  [unwired: 1 in, 3 out]
                n202 = case shown="True" w301 {
                  tunnel: [string[] ["Right", "Motor Control"] string[] ["Stop", "Hardware reset", "Software reset", "Motor Control"]] -> w304
                  frame False {
                  }
                  frame True {
                  }
                }
                n203 = for {
                  shift-right: [w311] -> w302
                  shift-left: w303 -> [w312]
                  tunnel: w304 -> [w310] mode=indexing
                  n204 = Enqueue Element(queue=w312, element=w310) -> (queue out=w311:refnum<queue>)  [unwired: 2 in, 2 out]
                }
                n205 = Select(t=TLB_MHL_States."Task 4b" ("Enum"), s=w301, f=TLB_MHL_States."Task 4a" ("Enum")) -> (s? t:f=w305:T6)
              }
              frame 11 {
                n206 = Flush Queue(queue=w313) -> ()  [unwired: 1 in, 3 out]
                n207 = Greater Or Equal?(x=w315, y=0.75) -> (x >= y?=w316:bool)
                n208 = case shown="False" w316 {
                  tunnel: [string[] ["Forward", "Motor control"] string[] ["Stop", "Hardware reset", "Software reset"]] -> w321
                  frame False {
                  }
                  frame True {
                  }
                }
                n209 = for {
                  shift-right: [w327] -> w319
                  shift-left: w320 -> [w328]
                  tunnel: w321 -> [w326] mode=indexing
                  n210 = Enqueue Element(queue=w328, element=w326) -> (queue out=w327:refnum<queue>)  [unwired: 2 in, 2 out]
                }
                n211 = Select(t=TLB_MHL_States."Task 4c" ("Enum"), s=w316, f=TLB_MHL_States."Task 4b" ("Enum")) -> (s? t:f=w318:T6)
              }
              frame 12 {
                n212 = Flush Queue(queue=w329) -> ()  [unwired: 1 in, 3 out]
                n213 = Less Or Equal?(x=w331, y=-0.65) -> (x <= y?=w332:bool)
                n214 = case shown="False" w332 {
                  tunnel: [string[] ["Left", "Motor Control"] string[] ["Stop", "Hardware reset", "Software reset", "Motor Control"]] -> w337
                  frame False {
                  }
                  frame True {
                  }
                }
                n215 = for {
                  shift-right: [w343] -> w334
                  shift-left: w335 -> [w344]
                  tunnel: w337 -> [w342] mode=indexing
                  n216 = Enqueue Element(queue=w344, element=w342) -> (queue out=w343:refnum<queue>)  [unwired: 2 in, 2 out]
                }
                n217 = Select(t=TLB_MHL_States."Task 4d" ("Enum"), s=w332, f=TLB_MHL_States."Task 4c" ("Enum")) -> (s? t:f=w336:T6)
              }
              frame 13 {
                n218 = Flush Queue(queue=w346) -> ()  [unwired: 1 in, 3 out]
                n219 = Or(x=w349, y=w348) -> (x .or. y?=w347:bool)
                n220 = case shown="True" w347 {
                  tunnel: [string[] ["Forward", "Ultrasonic Read", "Motor Control"] string[] ["Stop", "Hardware reset", "Software reset", "Motor Control"]] -> w353
                  frame False {
                  }
                  frame True {
                  }
                }
                n221 = for {
                  shift-right: [w359] -> w351
                  shift-left: w352 -> [w360]
                  tunnel: w353 -> [w358] mode=indexing
                  n222 = Enqueue Element(queue=w360, element=w358) -> (queue out=w359:refnum<queue>)  [unwired: 2 in, 2 out]
                }
                n223 = Select(t=TLB_MHL_States."Idle" ("Enum"), s=w347, f=TLB_MHL_States."Task 4d" ("Enum")) -> (s? t:f=w350:T6)
              }
              frame 5 {
                n224 = for {
                  shift-right: [w367] -> w362
                  shift-left: w363 -> [w368]
                  tunnel: string[] ["Software reset", "Hardware reset", "Motor Control"] -> [w366] mode=indexing
                  n225 = Enqueue Element(queue=w368, element=w366) -> (queue out=w367:refnum<queue>)  [unwired: 2 in, 2 out]
                }
              }
              frame 19 {
                n226 = Flush Queue(queue=w370) -> ()  [unwired: 1 in, 3 out]
                n227 = case shown="False" w371 {
                  tunnel: [string[] ["IR Sensor Read", "Calculate", "Forward", "Motor Control"] string[] ["Hardware reset", "Software reset", "Motor Control"]] -> w372
                  frame False {
                  }
                  frame True {
                  }
                }
                n228 = for {
                  shift-right: [w381] -> w374
                  shift-left: w373 -> [w382]
                  tunnel: w372 -> [w380] mode=indexing
                  n229 = Enqueue Element(queue=w382, element=w380) -> (queue out=w381:refnum<queue>)  [unwired: 2 in, 2 out]
                }
                n230 = Select(t=TLB_MHL_States."Idle" ("Enum"), s=w371, f=TLB_MHL_States."Wall follow mode" ("Enum")) -> (s? t:f=w376:T6)
              }
              frame 20 {
                n231 = Flush Queue(queue=w386) -> ()  [unwired: 1 in, 3 out]
                n232 = case shown="False" w384 {
                  tunnel: [string[] ["Ultrasonic read", "Forward", "NavX Correct", "Motor Control"] string[] ["Hardware reset", "Software reset", "Motor Control", ""]] -> w383
                  frame False {
                  }
                  frame True {
                  }
                }
                n233 = for {
                  shift-right: [w395] -> w388
                  shift-left: w387 -> [w396]
                  tunnel: w383 -> [w394] mode=indexing
                  n234 = Enqueue Element(queue=w396, element=w394) -> (queue out=w395:refnum<queue>)  [unwired: 2 in, 2 out]
                }
                n235 = Select(t=TLB_MHL_States."Idle" ("Enum"), s=w384, f=TLB_MHL_States."Drive Straight" ("Enum")) -> (s? t:f=w389:u16)
              }
              frame 18 {
                n236 = Flush Queue(queue=w398) -> ()  [unwired: 1 in, 3 out]
                n237 = case shown="True" w399 {
                  tunnel: [string[] ["Cam Acq"] string[] ["Hardware reset", "Software reset", "Cam Exit", ""]] -> w403
                  frame False {
                  }
                  frame True {
                  }
                }
                n238 = for {
                  shift-right: [w409] -> w401
                  shift-left: w402 -> [w410]
                  tunnel: w403 -> [w408] mode=indexing
                  n239 = Enqueue Element(queue=w410, element=w408) -> (queue out=w409:refnum<queue>)  [unwired: 2 in, 2 out]
                }
                n240 = Select(t=TLB_MHL_States."Idle" ("Enum"), s=w399, f=TLB_MHL_States."Acquire image" ("Enum")) -> (s? t:f=w400:T6)
              }
              frame 3 {
              }
              frame 4 {
                # ">>State Logic >>"
                n241 = for {
                  shift-right: [w419] -> w414
                  shift-left: w415 -> [w420]
                  tunnel: string[] ["Software reset", "Hardware reset", "Motor Control", "Cam Exit", "Pre-Exit", "Exit"] -> [w418] mode=indexing
                  n242 = Enqueue Element(queue=w420, element=w418) -> (queue out=w419:refnum<queue>)  [unwired: 2 in, 2 out]
                }
              }
              frame 0 {
              }
            }
          }
        }
        n243 = local write "GREEN LED State"(w103) -> ()
      }
      n244 = call <vilib>:"NavX Close.vi"("NavX Info In"=w28) -> ()  [unwired: 10 in, 1 out]
      n245 = while {
        shift-right: [w63] -> _
        shift-left: _ -> [w64]
        shift-right: [w62] -> _
        shift-left: _ -> [w61]
        stop <- w70 stop-if-true
        (unwired) TRUE
        # "LED Blinker Loop"
        n246 = case shown="\"OFF\", Default" "GREEN LED State" {
          tunnel: [FALSE TRUE w78] -> w66
          tunnel: w64 -> [_ _ w78]
          tunnel: [_ _ w79] -> w63
          frame "OFF", Default {
          }
          frame "ON" {
          }
          frame "BLINK" {
            n247 = Not(x=w78) -> (.not. x?=w79:bool)
          }
        }
        n248 = case shown="\"OFF\", Default" "RED LED State" {
          tunnel: [FALSE TRUE w74] -> w65
          tunnel: [_ _ w75] -> w62
          tunnel: w61 -> [_ _ w74]
          frame "OFF", Default {
          }
          frame "ON" {
          }
          frame "BLINK" {
            n249 = Not(x=w74) -> (.not. x?=w75:bool)
          }
        }
        n250 = local write "Green LED"(w66) -> ()
        n251 = local write "Red LED"(w65) -> ()
        n252 = call "FGV Stop.vi"("Init/Read/Write State"=States_for_Action_Engine."Read") -> ("Output node"=w70:bool)  [unwired: 2 in, 1 out]
        n253 = Wait (ms)(milliseconds to wait=u32 500) -> ()  [unwired: 1 out]
      }
      n254 = call <vilib>:"DIO Close.vi"("error in (no error)"=w20, "DIO Info In"=w26) -> ()  [unwired: 9 in, 1 out]
      n255 = call <vilib>:"DIO Close.vi"("error in (no error)"=w18, "DIO Info In"=w22) -> ()  [unwired: 9 in, 1 out]
      n256 = call <vilib>:"DIO Close.vi"("error in (no error)"=w8, "DIO Info In"=w13) -> ()  [unwired: 9 in, 1 out]
      n257 = call <vilib>:"DIO Close.vi"("error in (no error)"=w6, "DIO Info In"=w12) -> ()  [unwired: 9 in, 1 out]
      n258 = call <vilib>:"DIO Close.vi"("DIO Info In"=w4) -> ()  [unwired: 10 in, 1 out]
      n259 = Merge Errors "Merge Errors"(w54, w53) -> (w35:errorcluster)
      n260 = Merge Errors(w39, w35) -> (w29:errorcluster)
      n261 = Destroy User Event(user event=w57, error in=w29) -> ()  [unwired: 1 out]
      n262 = Destroy User Event(user event=w58, error in=w29) -> ()  [unwired: 1 out]
      n263 = Unregister For Events(event registration refnum=w49, error in=w29) -> ()  [unwired: 1 out]
      n264 = Release Queue(queue=w31, error in (no error)=w29) -> (error out=→"error out":errorcluster)  [unwired: 1 in, 2 out]
      n265 = Release Queue(queue=w48, error in (no error)=w29) -> ()  [unwired: 1 in, 3 out]
    }
    frame #2 {
      n266 = for {
        N: 20 -> [_]
        n267 = call "New motor Control integrated remodeled with PID.vi"("States"=enum16{"RESET ENCODER", "WRITE", "READ", "INIT"}."WRITE", "Target Speed"=T16 {"xTargetSpeed"=0.0, "yTargetSpeed"=0.0, "wTargetSpeed"=0.0}) -> ()  [unwired: 3 in, 2 out]
        n268 = Wait (ms)(milliseconds to wait=u32 10) -> ()  [unwired: 1 out]
      }
    }
  }
